vi "Test Step Name in Report.vi"(11 "Test Case In":refnum<class "Report CSV Content Test.lvclass">) -> (0 "error out":errorcluster, 3 "Test Case Out":refnum<class "Report CSV Content Test.lvclass">)   [LabVIEW 2020, in "Report CSV Content Test.lvclass"]
uses:
  Report CSV Content Test.lvclass
  4993e8ee-a06a-463a-9684-69129f64d5ce.vi
  source/Test Result Handler/TestStand Result Handler.lvclass
  source/Configuration/Configuration.lvclass
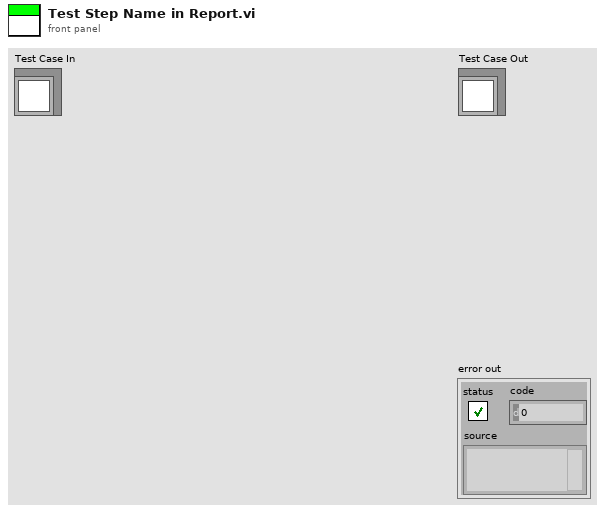
[diagram p1: front panel]
types:
  T1 = typedef "Astemes_CSVReportPlugin.lvlib/TestStand Result Handler.lvclass/TestStand Result.ctl" = cluster{"error in (no error)":errorcluster, "ReportText":string, "TS":cluster{"Index":i32, "BlockLevel":i32, "StartTime":dbl, "Id":i32, "StepType":string, "StepID":string, "StepGroup":string, "StepName":string}, "Status":string}
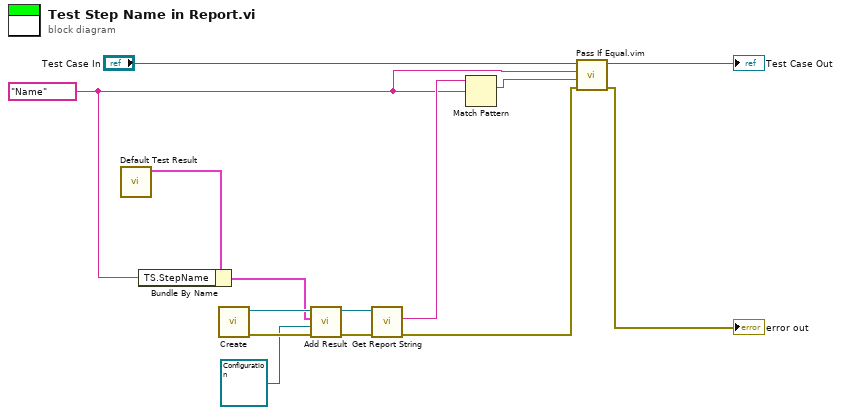
[diagram p0: block diagram]
diagram:
  w3 = "Name" ("Status")
  n1 = call "Default Test Result.vi"() -> ("TestStand Result"=w7:T1)  [unwired: 11 in]
  n2 = Bundle By Name(cluster=w7, "TS.StepName"=w3) -> (w6:T1)
  n3 = call "Create.vi"() -> ("error out"=w10:errorcluster, "Test Result Handler"=w11:refnum<class "TestStand Result Handler.lvclass">)  [unwired: 10 in]
  n4 = call "Add Result.vi"("error in (no error)"=w10, "Sequenc Context"=refnum<class "Configuration.lvclass"> refnum, "TestStand Result"=w6, "TestStand Result Handler In"=w11) -> ("error out"=w8:errorcluster, "TestStand Result Handler Out"=w9:refnum<class "TestStand Result Handler.lvclass">)  [unwired: 6 in]
  n5 = call "Get Report String.vi"("error in (no error)"=w8, "TestStand Result Handler In"=w9) -> ("error out"=w2:errorcluster, "Report Text"=w5:string)  [unwired: 8 in]
  n6 = Match Pattern(string=w5, regular expression=w3) -> (match substring=w4:string)  [unwired: 1 in, 3 out]
  n7 = call "Pass If Equal.vim"("error in (no error)"=w2, "Actual"=w4, "Expected"=w3, "LUnit Test Case In"="Test Case In") -> ("error out"=→"error out":errorcluster, "LUnit Test Case Out"=→"Test Case Out":refnum<class "Report CSV Content Test.lvclass">)  [unwired: 6 in]
